vi "SetAction.vi"(7 "Description":string, 8 "Command Info In":T2, 11 "Action":T1) -> (0 "Command Info Out":T2)   [LabVIEW 2018]
doc: "This template is useful for immediate subsystem actions that do not need deadband filtering\n\nBe sure to right-click and select New from Template and save with a new command name."
uses:
  <vilib>/Rock Robotics/WPI/Framework/Command Status Info.ctl
  <vilib>/Rock Robotics/WPI/Framework/Completion Status.ctl
  <vilib>/Rock Robotics/WPI/Framework/Completion Notifier.ctl
  Actions.ctl
  Implementation/LEDs Setpoints.ctl
  Implementation/LEDs Operations.ctl
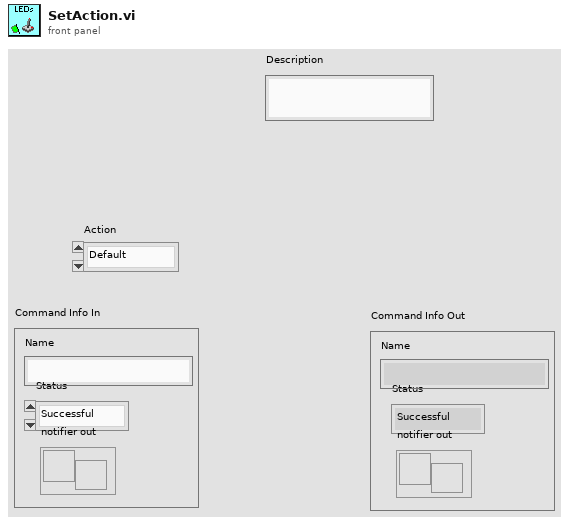
[diagram p1: front panel]
types:
  T1 = typedef "Actions.ctl" = enum16{"Default", "Hatch Triggered", "Lost Vision"}
  T2 = typedef "Command Status Info.ctl" = cluster{"Name":string, "Status":T3, "notifier out":T4}
  T3 = typedef "Completion Status.ctl" = enum16{"Successful", "Aborted", "Incomplete"}
  T4 = typedef "Completion Notifier.ctl" = refnum<notifier>
  T5 = typedef "LEDs Setpoints.ctl" = cluster{"Operation":T6, "Action":T1}
  T6 = typedef "LEDs Operations.ctl" = enum16{"Reserve", "Read Current", "Immediate"}
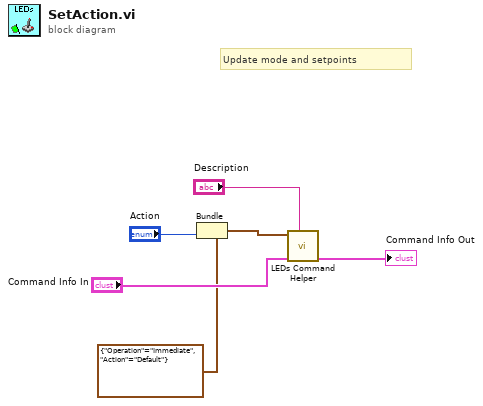
[diagram p0: block diagram]
diagram:
  # "Update mode and setpoints"
  n1 = Bundle(cluster=T5 {"Operation"=enum."Immediate", "Action"=enum."Default"} ("SubSystem Data"), "Action"="Action") -> (w2:T5)  [unwired: 1 in]
  n2 = call "LEDs Command Helper.vi"("Description"="Description", "Command Info In"="Command Info In", "SubSystem Data"=w2) -> ("Command Info Out"=→"Command Info Out":T2)  [unwired: 6 in, 2 out]
